vi "Tag Multi Channel.vi"(0 "Data in":i16[](array[numeric])=[0, 0, 0, 0], 1 "Tag Record":bool, 2 "TagData":T1, 3 "Input Valid":bool, 4 "Tag (I16)":i16=-32768) -> (7 "Data out":i16[](array[numeric]), 8 "Output Valid":bool, 9 "Pixel Overwritten":bool)   [LabVIEW 2014]
uses:
  Frametag Data.ctl
panel:
  # "Copyright 2014 Vidrio Technologies\nScanImage 5 software is licensed under the Apache License, Version 2.0 (the \"License\"); you may not use any files contained\nwithin the ScanImage 5 release except in compliance with the License. You may obtain a copy of the License at\n http://www.apache.org/licenses/LICENSE-2.0\nUnless required by applicable law or agreed to in writing, software distributed under the License is distributed on an\n\"AS IS\" BASIS, WITHOUT WARRANTIES OR CONDITIONS OF ANY KIND, either express or implied. See the License for the\n specific language governing permissions and limitations under the License."
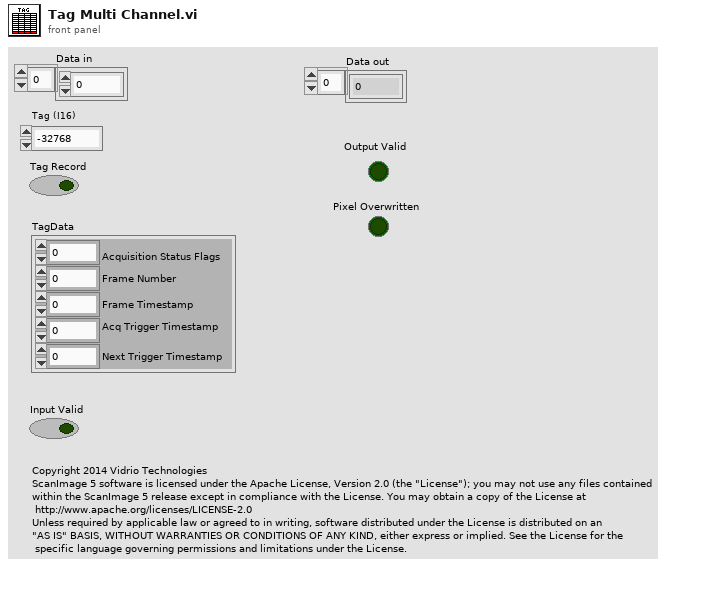
[diagram p1: front panel]
types:
  T1 = typedef "Frametag Data.ctl" = cluster{"Acquisition Status Flags":u16, "Frame Number":u32, "Frame Timestamp":u64, "Acq Trigger Timestamp":u64, "Next Trigger Timestamp":u64}
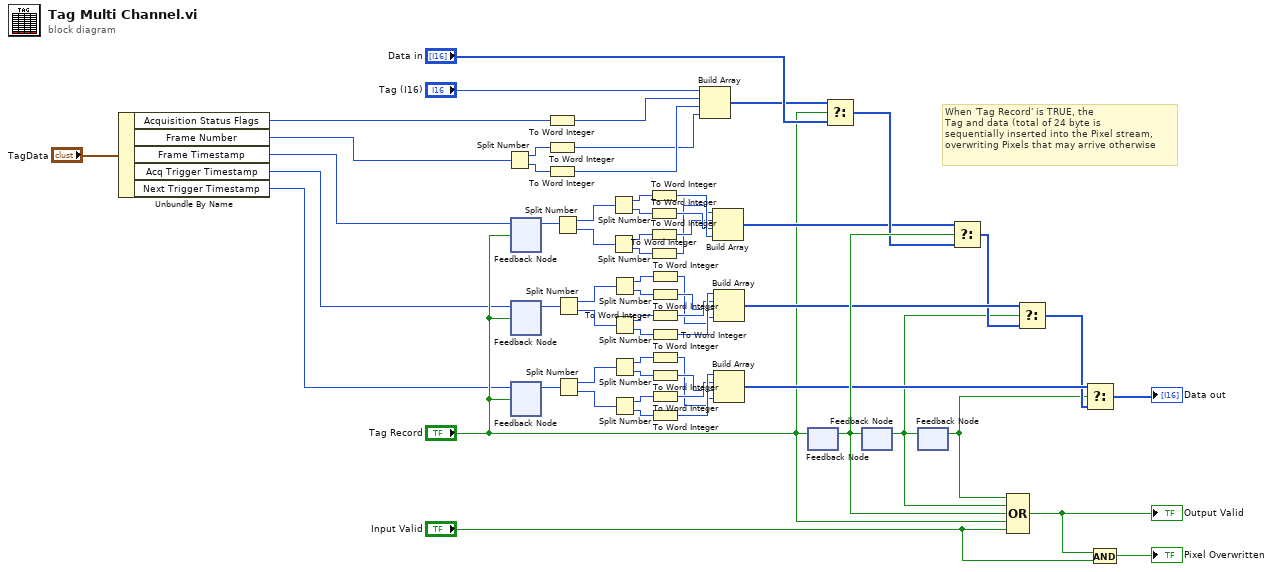
[diagram p0: block diagram]
diagram:
  # "When 'Tag Record' is TRUE, the\nTag and data (total of 24 byte is\nsequentially inserted into the Pixel stream,\noverwriting Pixels that may arrive otherwise"
  n1 = Unbundle By Name("TagData") -> ("Acquisition Status Flags"=w5:u16, "Frame Number"=w4:u32, "Frame Timestamp"=w3:u64, "Acq Trigger Timestamp"=w2:u64, "Next Trigger Timestamp"=w1:u64)
  n2 = Split Number(x=w4) -> (hi(x)=w59:u16, lo(x)=w58:u16)
  n3 = feedback-in #1(w3, "Tag Record") -> ()
  n4 = feedback #1() -> (w49:u64)  [unwired: 1 in]
  n5 = feedback #2() -> (w39:u64)  [unwired: 1 in]
  n6 = feedback-in #2(w2, "Tag Record") -> ()
  n7 = feedback #3() -> (w24:u64)  [unwired: 1 in]
  n8 = feedback-in #3(w1, "Tag Record") -> ()
  n9 = To Word Integer(number=w5) -> (16bit integer=w9:i16)
  n10 = To Word Integer(number=w59) -> (16bit integer=w7:i16)
  n11 = To Word Integer(number=w58) -> (16bit integer=w8:i16)
  n12 = Split Number(x=w49) -> (hi(x)=w55:u32, lo(x)=w50:u32)
  n13 = Split Number(x=w39) -> (hi(x)=w45:u32, lo(x)=w40:u32)
  n14 = Split Number(x=w24) -> (hi(x)=w29:u32, lo(x)=w34:u32)
  n15 = Split Number(x=w55) -> (hi(x)=w54:u16, lo(x)=w53:u16)
  n16 = Split Number(x=w50) -> (hi(x)=w51:u16, lo(x)=w52:u16)
  n17 = Split Number(x=w45) -> (hi(x)=w44:u16, lo(x)=w43:u16)
  n18 = Split Number(x=w40) -> (hi(x)=w41:u16, lo(x)=w42:u16)
  n19 = Split Number(x=w29) -> (hi(x)=w30:u16, lo(x)=w31:u16)
  n20 = Split Number(x=w34) -> (hi(x)=w33:u16, lo(x)=w32:u16)
  n21 = To Word Integer(number=w54) -> (16bit integer=w22:i16)
  n22 = To Word Integer(number=w53) -> (16bit integer=w21:i16)
  n23 = To Word Integer(number=w51) -> (16bit integer=w20:i16)
  n24 = To Word Integer(number=w52) -> (16bit integer=w19:i16)
  n25 = To Word Integer(number=w44) -> (16bit integer=w15:i16)
  n26 = To Word Integer(number=w43) -> (16bit integer=w16:i16)
  n27 = To Word Integer(number=w41) -> (16bit integer=w17:i16)
  n28 = To Word Integer(number=w42) -> (16bit integer=w18:i16)
  n29 = To Word Integer(number=w30) -> (16bit integer=w11:i16)
  n30 = To Word Integer(number=w31) -> (16bit integer=w12:i16)
  n31 = To Word Integer(number=w33) -> (16bit integer=w13:i16)
  n32 = To Word Integer(number=w32) -> (16bit integer=w14:i16)
  n33 = Build Array("Tag (I16)", w9, w8, w7) -> (w60:i16[])
  n34 = Build Array(w19, w20, w21, w22) -> (w38:i16[])
  n35 = Build Array(w18, w17, w16, w15) -> (w37:i16[])
  n36 = Build Array(w14, w13, w12, w11) -> (w35:i16[])
  n37 = feedback-in #4("Tag Record") -> ()
  n38 = feedback #4() -> (w47:bool)  [unwired: 1 in]
  n39 = Select(t=w60, s="Tag Record", f="Data in") -> (s? t:f=w46:i16[])
  n40 = feedback #5() -> (w26:bool)  [unwired: 1 in]
  n41 = feedback-in #5(w47) -> ()
  n42 = feedback #6() -> (w25:bool)  [unwired: 1 in]
  n43 = feedback-in #6(w26) -> ()
  n44 = Select(t=w38, s=w47, f=w46) -> (s? t:f=w36:i16[])
  n45 = Compound Arithmetic op=OR(w25, w26, w47, "Tag Record", "Input Valid") -> (w48:bool)
  "Output Valid" <- w48
  n46 = Select(t=w37, s=w26, f=w36) -> (s? t:f=w28:i16[])
  n47 = Select(t=w35, s=w25, f=w28) -> (s? t:f=→"Data out":i16[])
  n48 = And(x=w48, y="Input Valid") -> (x .and. y?=→"Pixel Overwritten":bool)
